vi "PDE_Error Handler.vi"(8 "error in (no error)":errorcluster, 11 "PDE error":T1) -> (0 "error out":errorcluster)   [LabVIEW 2017, in "NI_PDE.lvlib"]
uses:
  <vilib>/gmath/NI_PDE.lvlib
  <vilib>/gmath/pde.llb/Common/PDE_Error.ctl
panel:
  in  "source":string="PDE Solver"
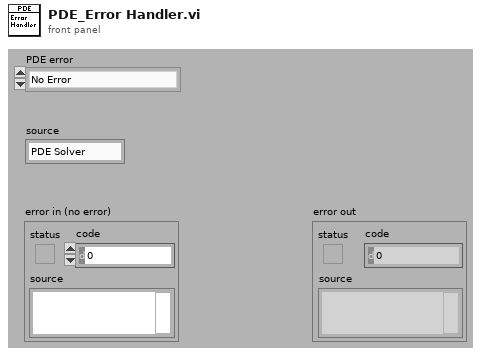
[diagram p1: front panel]
types:
  T1 = typedef "NI_PDE.lvlib/PDE_Error.ctl" = enum16{"No Error", "k is zero", "End point <= start point", "# of time steps < 2", "# of spatial points < 3", "# of grid < 1 for FEM", "# of boundary < 3 for FEM", "Incompatible RHS size", "Incompatible BC size", "Incompatible IC size", "PDE class conflict", "RHS class conflict", "Domain class conflict", "BC class conflict", "IC class conflict"}
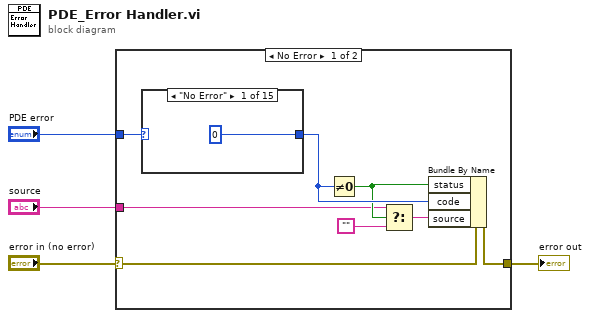
[diagram p0: block diagram]
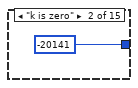
[diagram p2: hidden frame]
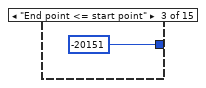
[diagram p3: hidden frame]
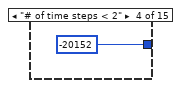
[diagram p4: hidden frame]
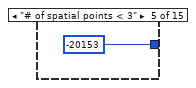
[diagram p5: hidden frame]
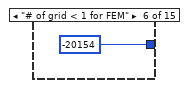
[diagram p6: hidden frame]
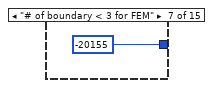
[diagram p7: hidden frame]
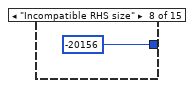
[diagram p8: hidden frame]
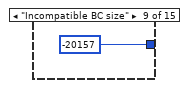
[diagram p9: hidden frame]
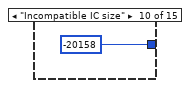
[diagram p10: hidden frame]
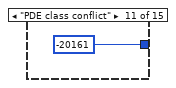
[diagram p11: hidden frame]
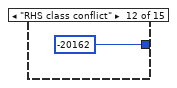
[diagram p12: hidden frame]
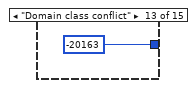
[diagram p13: hidden frame]
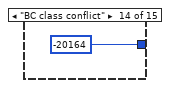
[diagram p14: hidden frame]
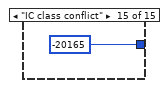
[diagram p15: hidden frame]
diagram:
  n1 = case shown="No Error" "error in (no error)" {
    selector: "error in (no error)" -> [w11 w28]
    tunnel: [w10 w28] -> w3
    tunnel: "PDE error" -> [w12 _]
    tunnel: "source" -> [w7 _]
    frame No Error {
      n2 = case shown="\"No Error\"" w12 {
        tunnel: [0 -20141 -20151 -20152 -20153 -20154 -20155 -20156 -20157 -20158 -20161 -20162 -20163 -20164 -20165] -> w9
        frame "No Error" {
        }
        frame "k is zero" {
        }
        frame "End point <= start point" {
        }
        frame "# of time steps < 2" {
        }
        frame "# of spatial points < 3" {
        }
        frame "# of grid < 1 for FEM" {
        }
        frame "# of boundary < 3 for FEM" {
        }
        frame "Incompatible RHS size" {
        }
        frame "Incompatible BC size" {
        }
        frame "Incompatible IC size" {
        }
        frame "PDE class conflict" {
        }
        frame "RHS class conflict" {
        }
        frame "Domain class conflict" {
        }
        frame "BC class conflict" {
        }
        frame "IC class conflict" {
        }
      }
      n3 = Not Equal To 0?(x=w9) -> (x != 0?=w8:bool)
      n4 = Select(t=w7, s=w8, f="") -> (s? t:f=w6:string)
      n5 = Bundle By Name(cluster=w11, "status"=w8, "code"=w9, "source"=w6) -> (w10:errorcluster)
    }
    frame Error {
    }
  }
  "error out" <- w3
